vi "Write State.vi"(8 "error in (no error)":errorcluster, 10 "State":enum16{"GoToBallKeeper", "Kick", "Exit"}(ring), 11 "GoalKickKeeperTacticVSS in":refnum<class "GoalKickKeeperTacticVSS.lvclass">) -> (0 "error out":errorcluster, 3 "GoalKickKeeperTacticVSS out":refnum<class "GoalKickKeeperTacticVSS.lvclass">)   [LabVIEW 2023, in "GoalKickKeeperTacticVSS.lvclass"]
uses:
  GoalKickKeeperTacticVSS.lvclass
  GoalKickKeeperTacticVSS.lvclass/GoalKickKeeperTacticVSS.ctl
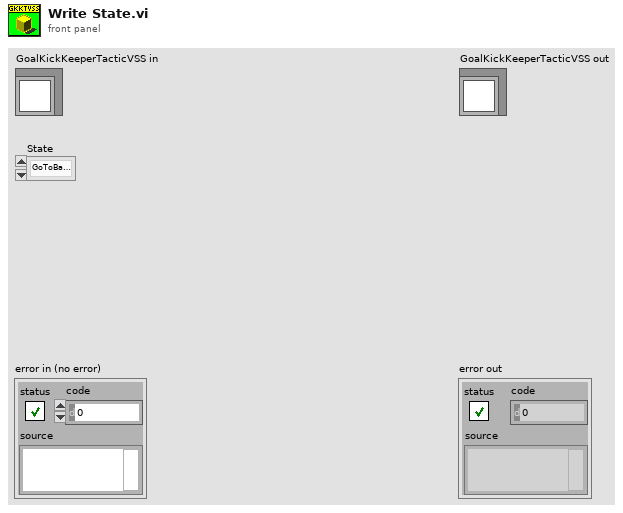
[diagram p1: front panel]
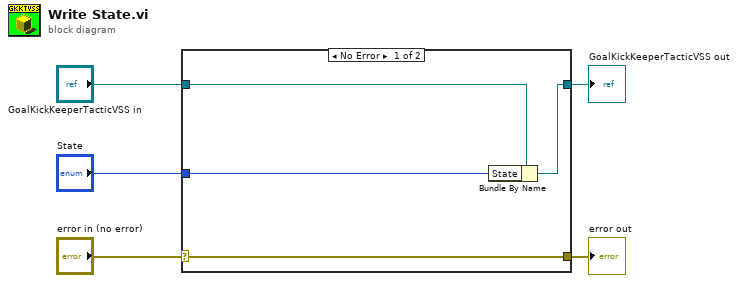
[diagram p0: block diagram]
diagram:
  n1 = case shown="No Error" "error in (no error)" {
    selector: "error in (no error)" -> [w9 w10]
    tunnel: [w9 w10] -> w4
    tunnel: [w7 w11] -> w2
    tunnel: "GoalKickKeeperTacticVSS in" -> [w8 w11]
    tunnel: "State" -> [w6 _]
    frame No Error {
      n2 = Bundle By Name(cluster=w8, "State"=w6) -> (w7:refnum<class "GoalKickKeeperTacticVSS.lvclass">)
    }
    frame Error {
    }
  }
  "error out" <- w4
  "GoalKickKeeperTacticVSS out" <- w2
